vi "GetTabCtrlRefGen.vi"(8 "ErrorIn(No Error)":errorcluster caption="entrée d'erreur (pas d'erreur)", 11 "CommandRef":refnum<vi>) -> (0 "sortie d'erreur":errorcluster, 2 "ControlsRefs":refnum<vi>[](array[refnum]), 3 "ControlsNames":string[](array[string]))   [LabVIEW 2010]
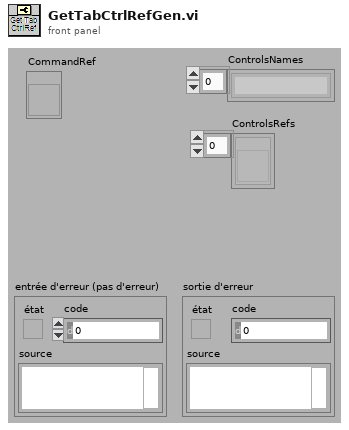
[diagram p1: front panel]
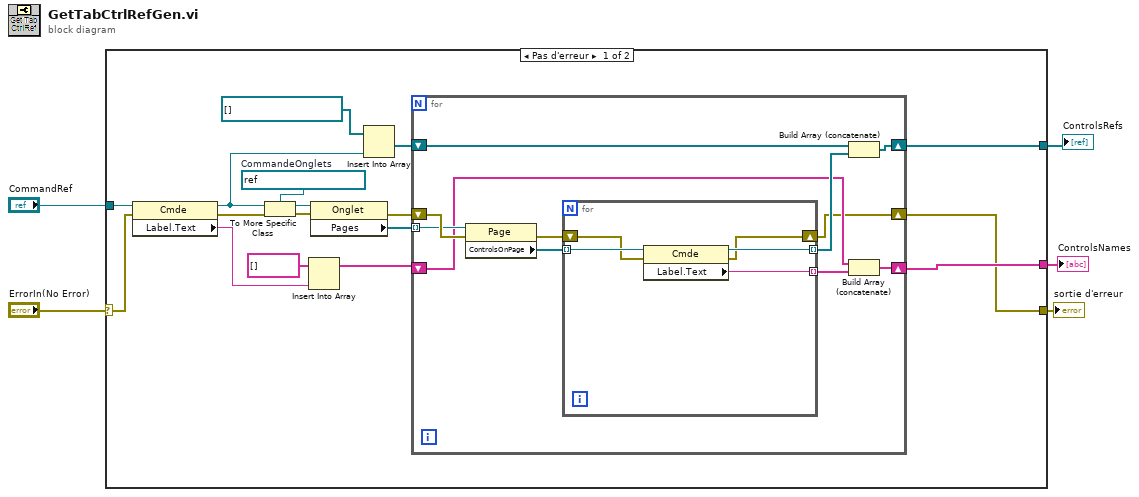
[diagram p0: block diagram]
diagram:
  n1 = case shown="Pas d'erreur" "ErrorIn(No Error)" {
    selector: "ErrorIn(No Error)" -> [w13 w39]
    tunnel: [w6 w39] -> w4
    tunnel: "CommandRef" -> [w15 _]
    tunnel: [w8 _] -> w2
    tunnel: [w7 _] -> w1
    frame No Error {
      w20 = refnum<vi> refnum  # CommandeOnglets
      n2 = property class="Cmde"(reference=w15, error in=w13) -> (reference out=w14:refnum<vi>, error out=w12:errorcluster, "Label.Text"=w10:string)
      n3 = To More Specific Class(target class=w20, reference=w14, error in=w12) -> (specific class reference=w21:refnum<vi>, error out=w22:errorcluster)
      n4 = Insert Into Array(array=string[] [] ("tableau"), new element=w10) -> (w11:string[])  [unwired: 1 in]
      n5 = property class="Onglet"(reference=w21, error in=w22) -> (error out=w18:errorcluster, "Pages"=w19:refnum<vi>[])  [unwired: 1 out]
      n6 = Insert Into Array(array=refnum<vi>[] [], new element=w14) -> (w17:refnum<vi>[])  [unwired: 1 in]
      n7 = for {
        tunnel: w19 -> [w30] mode=indexing
        shift-right: [w27] -> w8
        shift-left: w17 -> [w29]
        shift-right: [w25] -> w7
        shift-left: w11 -> [w24]
        shift-right: [w23] -> w6
        shift-left: w18 -> [w32]
        n8 = property class="Page"(reference=w30, error in=w32) -> (error out=w31:errorcluster, "ControlsOnPage"=w33:refnum<vi>[])  [unwired: 1 out]
        n9 = for {
          tunnel: w33 -> [w38] mode=indexing
          tunnel: [w37] -> w28 mode=indexing
          tunnel: [w36] -> w26 mode=indexing
          shift-right: [w34] -> w23
          shift-left: w31 -> [w35]
          n10 = property class="Cmde"(reference=w38, error in=w35) -> (reference out=w37:refnum<vi>, error out=w34:errorcluster, "Label.Text"=w36:string)
        }
        n11 = Build Array (concatenate)(w29, w28) -> (w27:refnum<vi>[])
        n12 = Build Array (concatenate)(w24, w26) -> (w25:string[])
      }
    }
    frame Error {
    }
  }
  "sortie d'erreur" <- w4
  "ControlsRefs" <- w2
  "ControlsNames" <- w1
